vi "TCP Buffered Write.vi"(8 "error in (no error)":errorcluster, 9 "read/write info":T1={"bytes to read"=0, "timeout ms"=25000, "read mode"=enum."line", "line separator"="\n"}, 10 "data in":string, 11 "connection ID":refnum<k5>) -> (0 "error out":errorcluster, 2 "bytes written":i32, 3 "connection ID out":refnum<k5>)   [LabVIEW 2015]
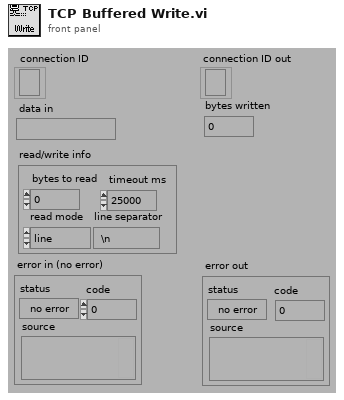
[diagram p1: front panel]
types:
  T1 = cluster{"bytes to read":i32, "timeout ms":i32, "read mode":enum16{"normal", "line", "buffered"}, "line separator":string}
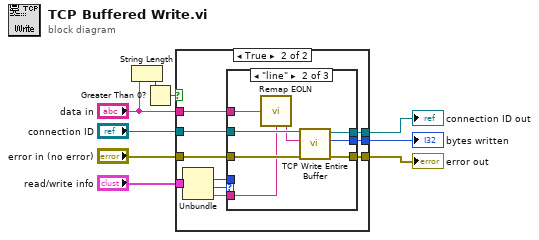
[diagram p0: block diagram]
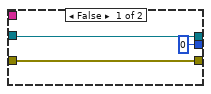
[diagram p2: hidden frame]
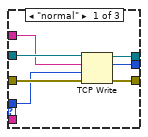
[diagram p3: hidden frame]
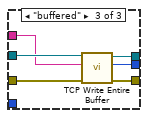
[diagram p4: hidden frame]
diagram:
  n1 = String Length(string="data in") -> (length=w2:i32)
  n2 = Greater Than 0?(x=w2) -> (x > 0?=w1:bool)
  n3 = case shown="True" w1 {
    tunnel: [w11 w22] -> w4
    tunnel: "data in" -> [_ w20]
    tunnel: [0 ("bytes written") w18] -> w5
    tunnel: "error in (no error)" -> [w11 w17]
    tunnel: [w12 w16] -> w7
    tunnel: "connection ID" -> [w12 w15]
    tunnel: "read/write info" -> [_ w13]
    frame False {
    }
    frame True {
      n4 = Unbundle(w13) -> ("timeout ms"=w19:i32, "read mode"=w14:enum16{"normal", "line", "buffered"}, "line separator"=w21:string)  [unwired: 1 out]
      n5 = case shown="\"line\"" w14 {
        tunnel: w15 -> [w29 w37 w43]
        tunnel: [w28 w36 w42] -> w16
        tunnel: w17 -> [w27 w35 w41]
        tunnel: [w26 w34 w40] -> w22
        tunnel: [w25 w33 w39] -> w18
        tunnel: w19 -> [w24 _ _]
        tunnel: w20 -> [w23 w32 w38]
        tunnel: w21 -> [_ w30 _]
        frame "normal" {
          n6 = TCP Write(connection ID=w29, data in=w23, error in (no error)=w27, 9:w24) -> (connection ID out=w28:refnum<k5>, bytes written=w25:i32, error out=w26:errorcluster)
        }
        frame "line" {
          n7 = call "Remap EOLN.vi"("string in"=w32, "line separator (\\r\\n)"=w30) -> ("string out"=w31:string)
          n8 = call "TCP Write Entire Buffer.vi"("error in (no error)"=w35, "data in"=w31, "connection ID"=w37) -> ("error out"=w34:errorcluster, "bytes written"=w33:i32, "connection ID out"=w36:refnum<k5>)  [unwired: 6 in]
        }
        frame "buffered" {
          n9 = call "TCP Write Entire Buffer.vi"("error in (no error)"=w41, "data in"=w38, "connection ID"=w43) -> ("error out"=w40:errorcluster, "bytes written"=w39:i32, "connection ID out"=w42:refnum<k5>)  [unwired: 6 in]
        }
      }
    }
  }
  "bytes written" <- w5
  "connection ID out" <- w7
  "error out" <- w4
